vi "TSLIN_SetData.vi"(8 "错误输入（无错误）":errorcluster, 10 "Set":T1={"硬件类型"=3, "硬件子类型"=10, "AHwChannel"=0, "AAppChannel"=0, "ABaudrateKbps"=250.0, "AProtocol"=2} {"AProtocol" items=["Lin_Protocol_13", "Lin_Protocol_20", "Lin_Protocol_21", "Lin_Protocol_J2602"]; "AAppChannel" items=["CHN1", "CHN2", "CHN3", "CHN4", "CHN5", "CHN6", "CHN7", "CHN8", "CHN9", "CHN10", "CHN11", "CHN12", "CHN13", "CHN14", "CHN15", "CHN16", "CHN17", "CHN18", "CHN19", "CHN20", "CHN21", "CHN22", "CHN23", "CHN24", "CHN25", "CHN26", "CHN27", "CHN28", "CHN29", "CHN30", "CHN31", "CHN32"]; "AHwChannel" items=["CHN1", "CHN2", "CHN3", "CHN4", "CHN5", "CHN6", "CHN7", "CHN8", "CHN9", "CHN10", "CHN11", "CHN12", "CHN13", "CHN14", "CHN15", "CHN16", "CHN17", "CHN18", "CHN19", "CHN20", "CHN21", "CHN22", "CHN23", "CHN24", "CHN25", "CHN26", "CHN27", "CHN28", "CHN29", "CHN30", "CHN31", "CHN32"]; "硬件子类型" items=["BUS_UNKNOWN_TYPE", "TSCAN_PRO_4", "TSCAN_LITE_2", "TSCANMini", "TSLinMini", "TSCANFDmini", "TSCAN_LIN_IO_2", "TSCAN_LITE_2", "TSCANLIN", "TSCAN_FD_Mini_1", "TSLIN1026"]; "硬件类型" items=["BUS_UNKNOWN_TYPE", "TS_TCP_DEVICE", "XL_USB_DEVICE", "TS_USB_DEVICE", "PEAK_USB_DEVICE", "KVASER_USB_DEVICE", "ZLG_USB_DEVICE", "ICS_USB_DEVICE", "TS_TC1005_DEVICE"]}, 11 "路径输入":path) -> (0 "错误输出":errorcluster, 3 "路径输出":path, 4 "Set_Baudrated_Successfully":bool, 6 "Mapping_Successfully":bool)   [LabVIEW 2019]
panel:
  # "用N路can通道，设置N路CAN通道"
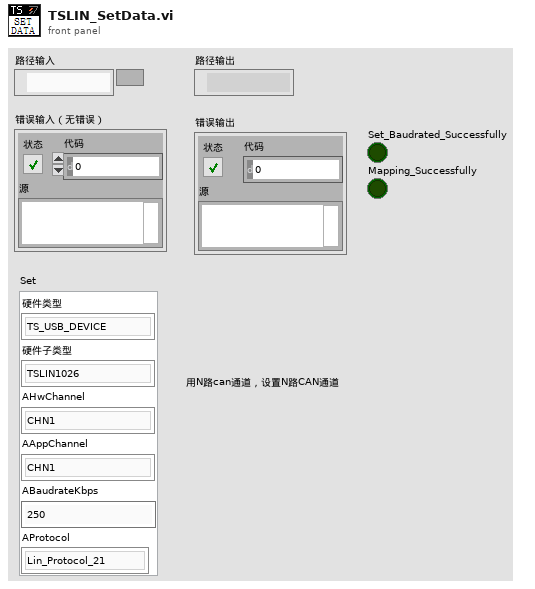
[diagram p1: front panel]
types:
  T1 = cluster{"硬件类型":i32, "硬件子类型":i32, "AHwChannel":i32, "AAppChannel":i32, "ABaudrateKbps":sgl, "AProtocol":i32}
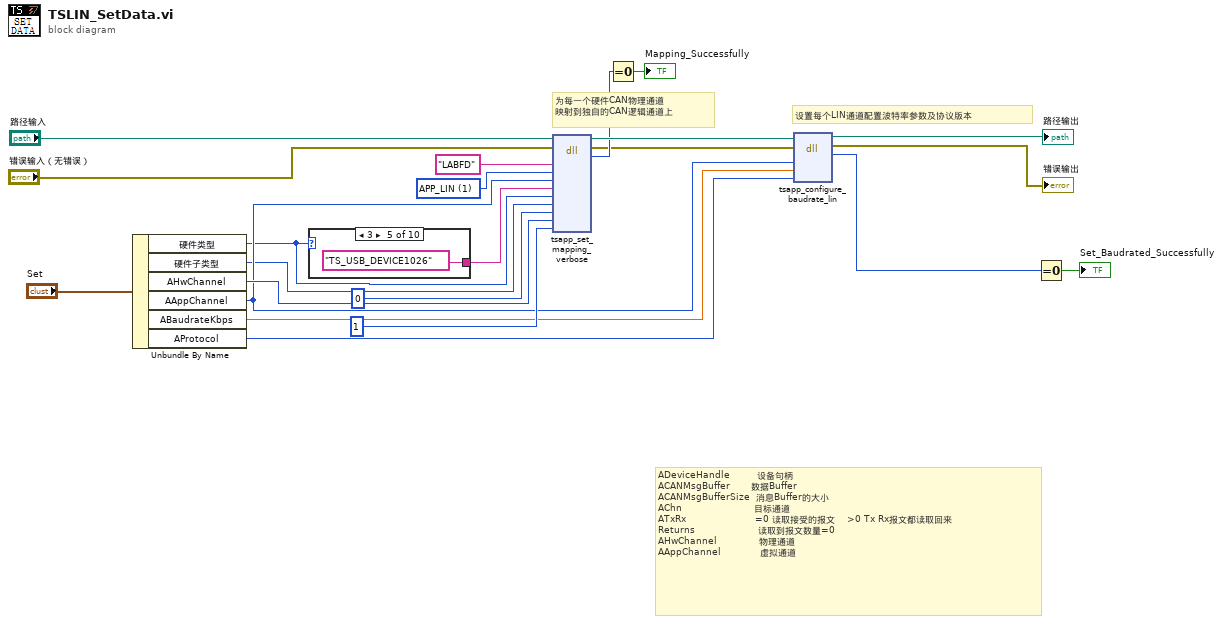
[diagram p0: block diagram]
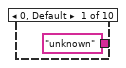
[diagram p2: hidden frame]
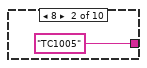
[diagram p3: hidden frame]
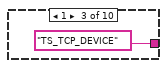
[diagram p4: hidden frame]
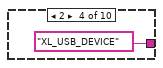
[diagram p5: hidden frame]
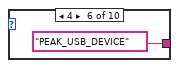
[diagram p6: hidden frame]
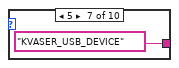
[diagram p7: hidden frame]
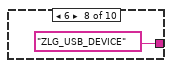
[diagram p8: hidden frame]
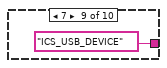
[diagram p9: hidden frame]
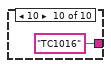
[diagram p10: hidden frame]
diagram:
  w20 = 1 items=["APP_CAN", "APP_LIN"] ("AAppChannelType")
  # "设置每个LIN通道配置波特率参数及协议版本"
  # "ADeviceHandle         设备句柄\nACANMsgBuffer       数据Buffer\nACANMsgBufferSize  消息Buffer的大小\nAChn                        目标通道\nATxRx                       =0 读取接受的报文    >0 Tx Rx报文都读取回来\nReturns                     读取到报文数量=0\nAHwChannel              物理通道\nAAppChannel             虚拟通道"
  # "为每一个硬件CAN物理通道\n映射到独自的CAN逻辑通道上"
  n1 = Unbundle By Name("Set") -> ("硬件类型"=w1:i32, "硬件子类型"=w2:i32, "AHwChannel"=w6:i32, "AAppChannel"=w5:i32, "ABaudrateKbps"=w4:sgl, "AProtocol"=w3:i32)
  n2 = case shown="3" w1 {
    tunnel: ["unknown" ("AHardwareName") "TC1005" ("AHardwareName") "TS_TCP_DEVICE" ("AHardwareName") "XL_USB_DEVICE" ("AHardwareName") "TS_USB_DEVICE1026" ("AHardwareName") "PEAK_USB_DEVICE" ("AHardwareName") "KVASER_USB_DEVICE" ("AHardwareName") "ZLG_USB_DEVICE" ("AHardwareName") "ICS_USB_DEVICE" ("AHardwareName") "TC1016" ("AHardwareName")] -> w19
    frame 0, Default {
    }
    frame 8 {
    }
    frame 1 {
    }
    frame 2 {
    }
    frame 3 {
    }
    frame 4 {
    }
    frame 5 {
    }
    frame 6 {
    }
    frame 7 {
    }
    frame 10 {
    }
  }
  n3 = dll-call lib="PTH2Habs CUsers\nAdministratorDesktopTS_Can通讯PathTSMaster.dll" fn="tsapp_set_mapping_verbose"(path in="路径输入", error in="错误输入（无错误）", "FAPppName"="LABFD" ("AppName"), "AChnType"=w20, "FAppChannelIndex"=w5, "AHWDeviceName"=w19, "AHWDeviceType"=w1, "AHWDeviceSubType"=w2, "AldHW"=0, "AldHWChn"=w6, "FMappingDisabled"=u32 1) -> (path out=w22:path, error out=w12:errorcluster, "tsapp_set_mapping_verbose"=w13:i32)  [unwired: 10 in]
  n4 = Equal To 0?(x=w13) -> (x = 0?=→"Mapping_Successfully":bool)
  n5 = dll-call lib="PTH2@abs EDemo同星TSCAN_V1.4_20220301ConfigTSMaster.dll" fn="tsapp_configure_baudrate_lin"(path in=w22, error in=w12, "ALdxChn"=w5, "ABaudrateKbps"=w4, "AProtocol"=w3) -> (path out=→"路径输出":path, error out=→"错误输出":errorcluster, "tsapp_configure_baudrate_can"=w14:i32)  [unwired: 4 in]
  n6 = Equal To 0?(x=w14) -> (x = 0?=→"Set_Baudrated_Successfully":bool)
